vi "hamamatsuReadToBuffer.vi"   [LabVIEW 2017]
uses:
  globalUtilities.vi
  globalDevices.vi
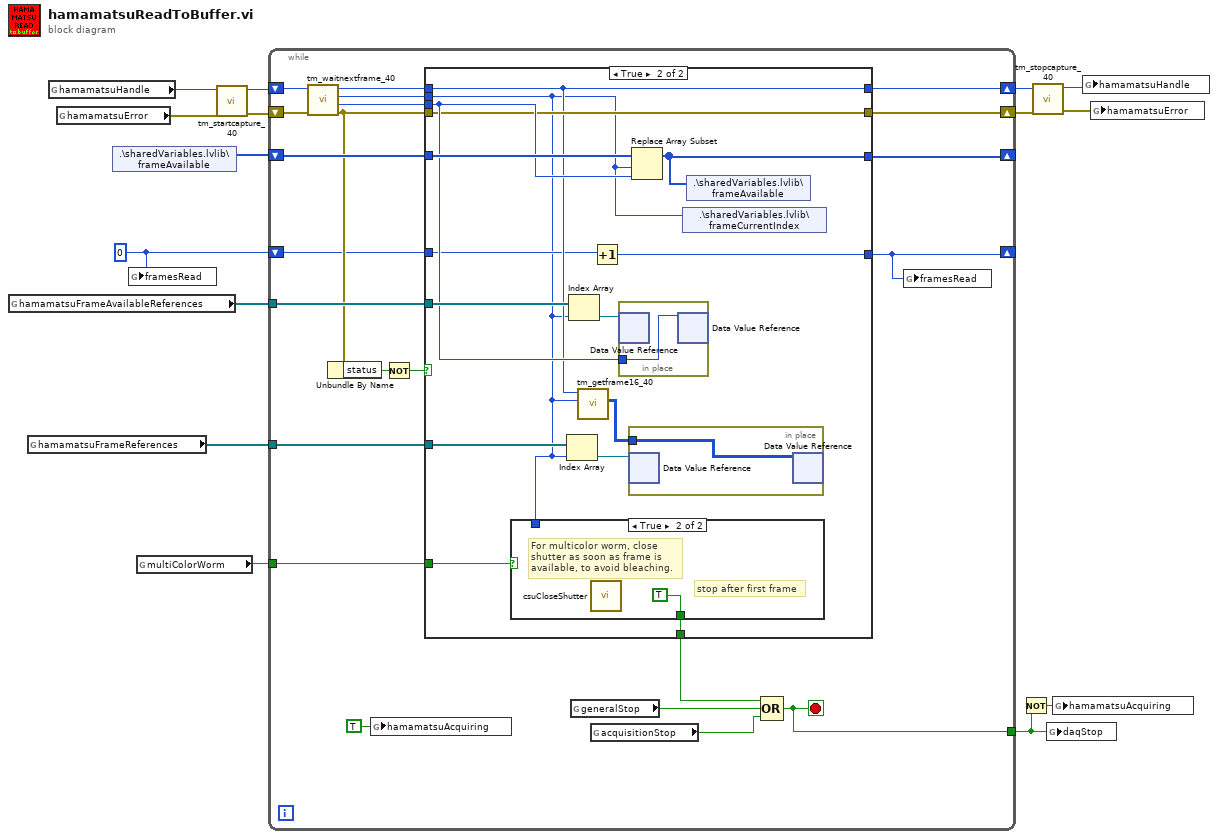
[diagram p0: block diagram]
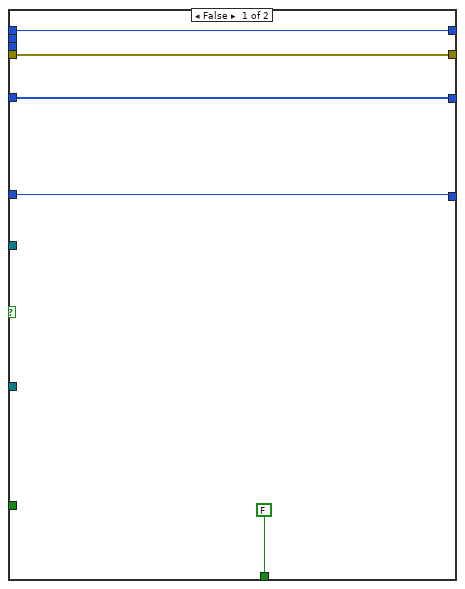
[diagram p2: hidden frame]
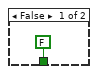
[diagram p3: hidden frame]
diagram:
  w1 = u32 0 ("framesRead")
  n1 = global read "globalDevices.vi" "hamamatsuFrameAvailableReferences"() -> (w3:refnum<data-value>[])
  n2 = global read "globalDevices.vi" "hamamatsuFrameReferences"() -> (w2:refnum<data-value>[])
  n3 = global read "globalDevices.vi" "hamamatsuHandle"() -> (w12:u32)
  n4 = global read "globalDevices.vi" "hamamatsuError"() -> (w11:errorcluster)
  n5 = shared-variable ".\\sharedVariables.lvlib\\frameAvailable"() -> (w5:i32[])  [unwired: 1 in, 1 out]
  n6 = global write "globalUtilities.vi" "framesRead"(w1) -> ()
  n7 = global read "globalUtilities.vi" "multiColorWorm"() -> (w4:bool)
  n8 = call <userlib>:"tm_startcapture_40.vi"("error in (no error)"=w11, "Handle in"=w12) -> ("error out"=w14:errorcluster, "Handle out"=w13:u32)  [unwired: 8 in]
  n9 = while {
    shift-right: [w26] -> w15
    shift-left: w14 -> [w36]
    shift-right: [w34] -> _
    shift-left: w5 -> [w35]
    tunnel: [w18] -> w7
    shift-right: [w25] -> w10
    shift-left: w13 -> [w37]
    tunnel: w4 -> [w32]
    tunnel: w3 -> [w31]
    tunnel: w2 -> [w29]
    shift-right: [w16] -> _
    shift-left: w1 -> [w17]
    stop <- w18 stop-if-true
    n10 = call <userlib>:"tm_waitnextframe_40.vi"("error in (no error)"=w36, "Handle in"=w37) -> ("error out"=w24:errorcluster, "Frame Count"=w27:i32, "Frame Index"=w30:i32, "Handle out"=w28:u32)  [unwired: 6 in]
    n11 = Unbundle By Name(w24) -> ("status"=w23:bool)
    n12 = global write "globalUtilities.vi" "hamamatsuAcquiring"(TRUE ("hamamatsuAcquiring")) -> ()
    n13 = Not(x=w23) -> (.not. x?=w22:bool)
    n14 = case shown="True" w22 {
      tunnel: w35 -> [w42 w57]
      tunnel: [w42 w56] -> w34
      tunnel: w32 -> [_ w55]
      tunnel: w31 -> [_ w54]
      tunnel: w30 -> [_ w43]
      tunnel: w29 -> [_ w52]
      tunnel: w28 -> [w40 w48]
      tunnel: w27 -> [_ w50]
      tunnel: w24 -> [w41 w49]
      tunnel: [w41 w49] -> w26
      tunnel: [w40 w48] -> w25
      tunnel: [FALSE w47] -> w21
      tunnel: w17 -> [w38 w46]
      tunnel: [w38 w45] -> w16
      frame False {
      }
      frame True {
        n15 = case shown="True" w55 {
          tunnel: w43 -> [_ _]
          tunnel: [FALSE TRUE] -> w47
          frame False {
          }
          frame True {
            # "stop after first frame"
            # "For multicolor worm, close\nshutter as soon as frame is\navailable, to avoid bleaching."
            n16 = call "csuCloseShutter.vi"() -> ()  [unwired: 16 in]
          }
        }
        n17 = Index Array(array=w52, index=w43) -> (element=w51:refnum<data-value>)
        n18 = Index Array(array=w54, index=w43) -> (element=w53:refnum<data-value>)
        n19 = call <userlib>:"tm_getframe16_40.vi"("Frame Index"=w43, "Handle in"=w48) -> ("Data"=w44:u16[][])  [unwired: 6 in, 3 out]
        n20 = Increment(x=w46) -> (x+1=w45:u32)
        n21 = in-place {
          in-place-border: w50 -> [w59]
          n22 = in-place-dvr #1(w53) -> ()  [unwired: 2 out]
          n23 = in-place-dvr #1(w59) -> ()  [unwired: 2 out]
        }
        n24 = in-place {
          in-place-border: w44 -> [w58]
          n25 = in-place-dvr #2(w51) -> ()  [unwired: 2 out]
          n26 = in-place-dvr #2(w58) -> ()  [unwired: 2 out]
        }
        n27 = Replace Array Subset(array=w57, new element=w50, index=w43) -> (w56:i32[])
        n28 = shared-variable ".\\sharedVariables.lvlib\\frameCurrentIndex"(w43) -> ()  [unwired: 1 in, 1 out]
        n29 = shared-variable ".\\sharedVariables.lvlib\\frameAvailable"(w56) -> ()  [unwired: 1 in, 1 out]
      }
    }
    n30 = global read "globalUtilities.vi" "generalStop"() -> (w20:bool)
    n31 = global read "globalUtilities.vi" "acquisitionStop"() -> (w19:bool)
    n32 = Compound Arithmetic op=OR(w21, w20, w19) -> (w18:bool)
    n33 = global write "globalUtilities.vi" "framesRead"(w16) -> ()
  }
  n34 = Not(x=w7) -> (.not. x?=w6:bool)
  n35 = call <userlib>:"tm_stopcapture_40.vi"("error in (no error)"=w15, "Handle in"=w10) -> ("error out"=w8:errorcluster, "Handle out"=w9:u32)  [unwired: 8 in]
  n36 = global write "globalUtilities.vi" "daqStop"(w7) -> ()
  n37 = global write "globalUtilities.vi" "hamamatsuAcquiring"(w6) -> ()
  n38 = global write "globalDevices.vi" "hamamatsuHandle"(w9) -> ()
  n39 = global write "globalDevices.vi" "hamamatsuError"(w8) -> ()
